vi "Lab1_WANG Zhenqiao.vi"() -> ()   [LabVIEW 2014]
uses:
  <vilib>/Utility/file.llb/Read From Spreadsheet File (string).vi
  <vilib>/Utility/file.llb/Write To Spreadsheet File (string).vi
panel:
  out "current speed":string
  out "appended array 2":string[](array[string])
  out "file output":path
  out "millisecond timer value":u32
  out "iteration":i32
  in  "file path (dialog if empty)":path
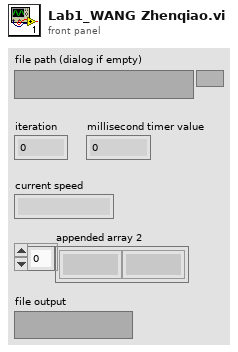
[diagram p1: front panel]
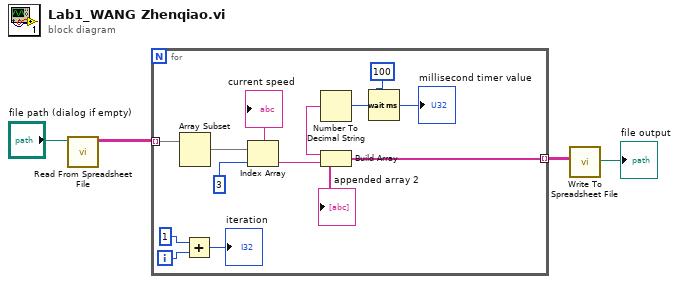
[diagram p0: block diagram]
diagram:
  n1 = call-poly <vilib>:"Read From Spreadsheet File.vi"("file path (dialog if empty)"="file path (dialog if empty)") -> ("all rows"=w2:string[][])  [unwired: 6 in, 4 out]
  n2 = for {
    tunnel: w2 -> [w8] mode=indexing
    tunnel: [w7] -> w1 mode=indexing
    i -> [w15]
    n3 = Array Subset(array=w8) -> (w12:string[])  [unwired: 2 in]
    n4 = Add(x=1, y=w15) -> (x+y=→"iteration":i32)
    n5 = Index Array(array=w12, index=3) -> (element=w6:string)
    "current speed" <- w6
    n6 = Wait (ms)(milliseconds to wait=u32 100) -> (millisecond timer value=w9:u32)
    "millisecond timer value" <- w9
    n7 = Number To Decimal String(number=w9) -> (decimal integer string=w5:string)  [unwired: 1 in]
    n8 = Build Array(w5, w6) -> (w7:string[])
    "appended array 2" <- w7
  }
  n9 = call-poly <vilib>:"Write To Spreadsheet File.vi"("2D data"=w1) -> ("new file path (Not A Path if cancelled)"=→"file output":path)  [unwired: 7 in]
